vi "Memory Map to Messages.vi"(4 "Smallest Write Command Size":u32(ring)=4 items=["256-bytes"=256, "128-bytes"=128, "64-bytes"=64, "32-bytes"=32, "16-bytes"=16, "8-bytes"=8, "4-bytes"=4], 5 "Erase Block Size":u32(ring)=1024 items=["1024-bytes"=1024, "512-bytes"=512, "256-bytes"=256, "128-bytes"=128, "64-bytes"=64, "32-bytes"=32, "16-bytes"=16, "8-bytes"=8], 6 "Largest Write Command Size":u32(ring)=256 items=["256-bytes"=256, "128-bytes"=128, "64-bytes"=64, "32-bytes"=32, "16-bytes"=16, "8-bytes"=8], 7 "Empty Range Thld":i32=8, 8 "error in":errorcluster, 10 "Check Memory Block Size":u32(ring)=16 items=["1024-bytes"=1024, "512-bytes"=512, "256-bytes"=256, "128-bytes"=128, "64-bytes"=64, "32-bytes"=32, "16-bytes"=16, "8-bytes"=8], 11 "base path":path=path "C:/SCU Flash Application/ODX File/C70/FlashDrvRAM.s19") -> (0 "Error Out":errorcluster, 1 "read memory list":cluster{"Address":i32, "Data":u8[]}[](array[cluster]) {"Address" format="%x"}, 2 "erase addresses":u32[](array[numeric]) format="%x", 3 "Messages":cluster{"Address":i32, "Data":u8[]}[](array[cluster]) {"Address" format="%.0x"; "Data" format="%.0x"})   [LabVIEW 2018]
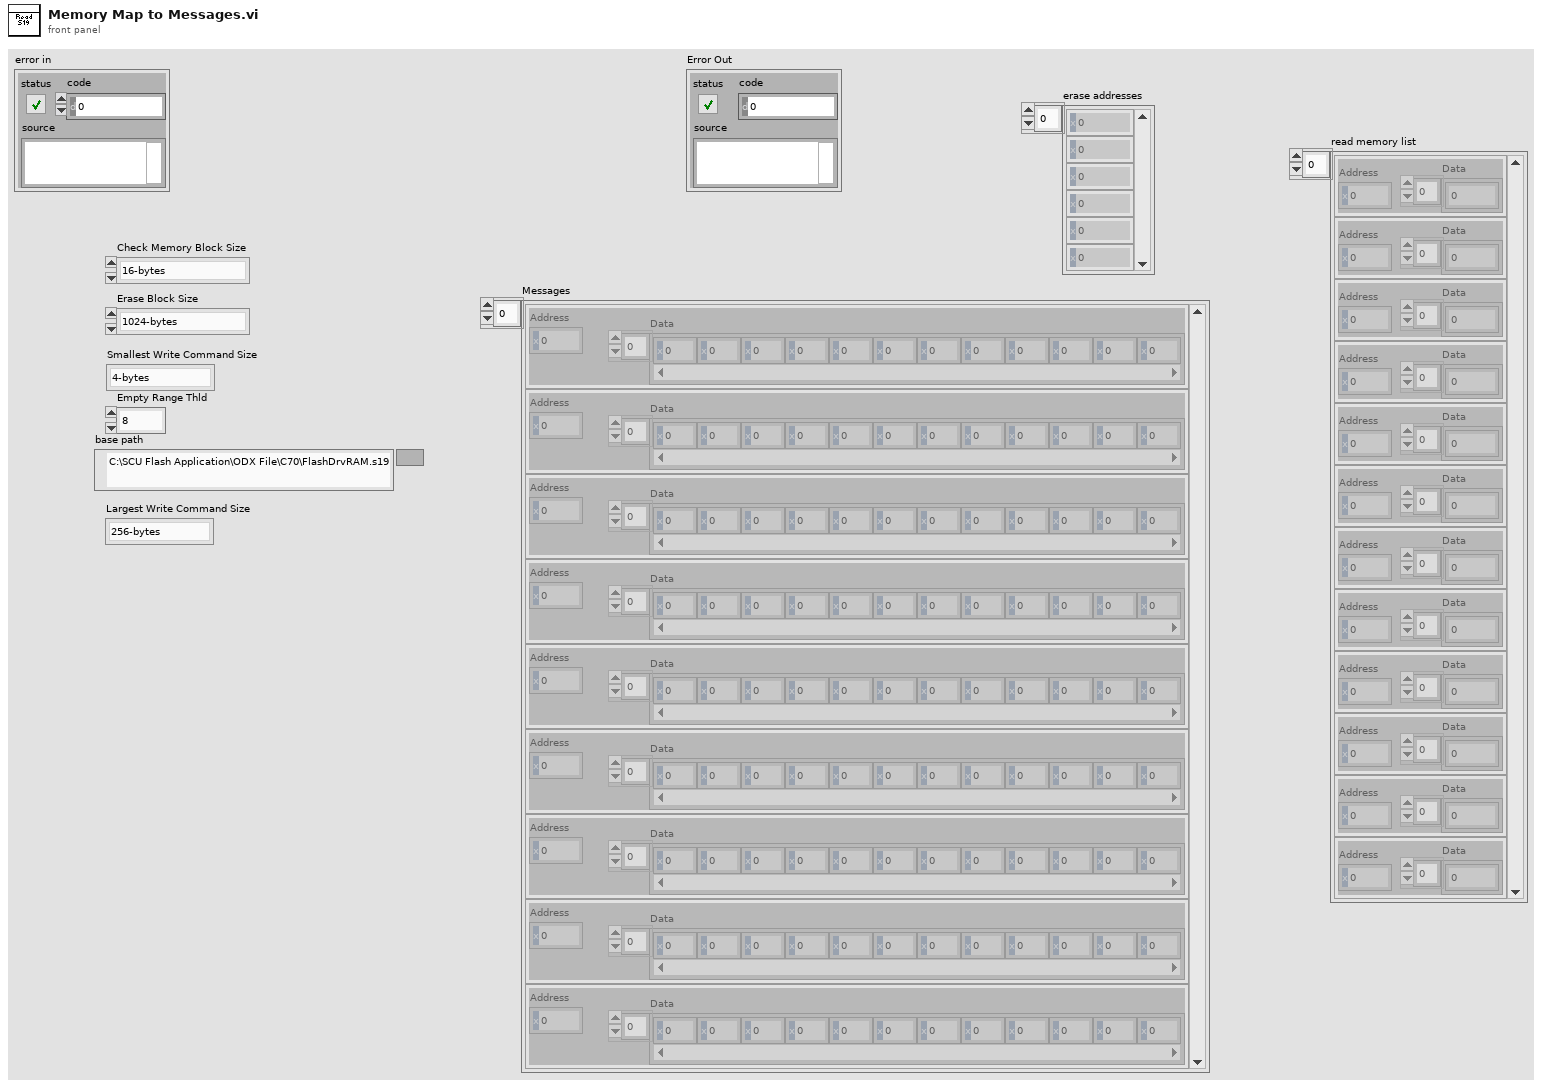
[diagram p1: front panel]
types:
  T1 = cluster{"Address":u32, "Data":u8[], "CheckSUM":u32}[]
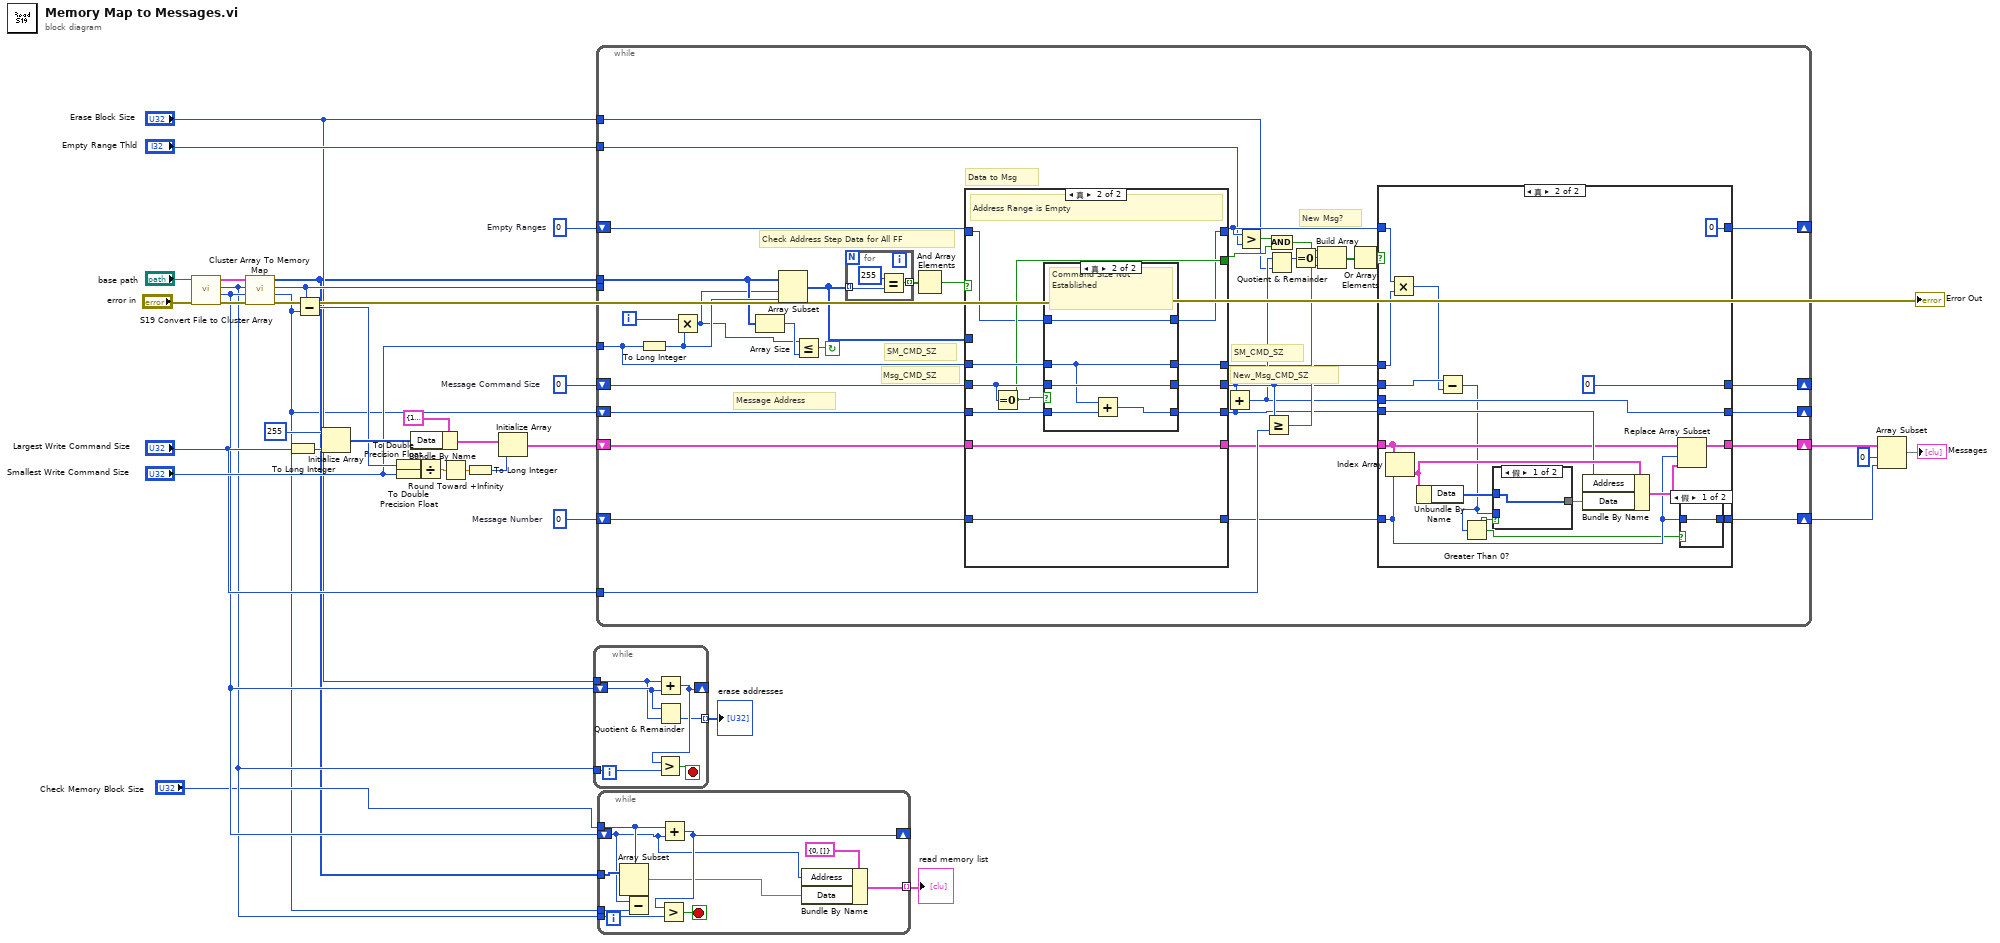
[diagram p0: block diagram]
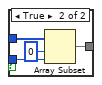
[diagram p3: hidden frame]
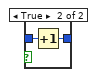
[diagram p4: hidden frame]
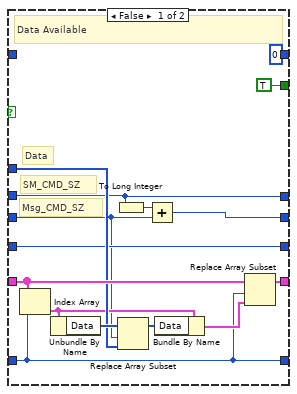
[diagram p5: hidden frame]
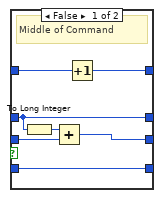
[diagram p6: hidden frame]
diagram:
  w19 = 0  # Empty Ranges
  w20 = 0  # Message Command Size
  w22 = 0  # Message Number
  n1 = call "S19 Convert File to Cluster Array.vi"("error in"="error in", "base path"="base path") -> ("Error Out"=→"Error Out":errorcluster, "Address Min"=w7:u32, "Address Max"=w6:u32, "数组"=w1:T1)  [unwired: 6 in]
  n2 = call "Cluster Array To Memory Map.vi"("Address Min in"=w7, "Address Max in"=w6, "Array in"=w1) -> ("Address Min out"=w3:u32, "Address Max out"=w10:u32, "Array out"=w4:u8[])  [unwired: 6 in]
  n3 = To Long Integer(number="Largest Write Command Size") -> (32bit integer=w34:i32)
  n4 = Subtract(x=w10, y=w3) -> (x-y=w29:u32)
  n5 = Initialize Array(u8 255 ("element"), w34) -> (w31:u8[])
  n6 = To Double Precision Float(number=w29) -> (double precision float=w25:dbl)
  n7 = To Double Precision Float(number="Smallest Write Command Size") -> (double precision float=w24:dbl)
  n8 = Bundle By Name(cluster=cluster{"Address":i32, "Data":u8[]} {"Address"=16777215, "Data"=[]} ("Line Data"), "Data"=w31) -> (w30:cluster{"Address":i32, "Data":u8[]})
  n9 = Divide(x=w25, y=w24) -> (x/y=w28:dbl)
  n10 = Round Toward +Infinity(x=w28) -> (ceil(x): smallest int >= x=w27:dbl)
  n11 = To Long Integer(number=w27) -> (32bit integer=w26:i32)
  n12 = Initialize Array(w30, w26) -> (w23:cluster{"Address":i32, "Data":u8[]}[])
  n13 = while {
    tunnel: [w38] -> w8 mode=indexing
    shift-right: [w39] -> _
    shift-left: w7 -> [w37]
    tunnel: w6 -> [w40]
    tunnel: "Erase Block Size" -> [w36]
    stop <- w41 stop-if-true
    n14 = Add(x=w36, y=w37) -> (x+y=w39:u32)
    n15 = Greater?(x=w39, y=w40) -> (0:w41:bool)
    n16 = Quotient & Remainder(x=w37, y=w36) -> (floor(x/y)=w38:u32)  [unwired: 1 out]
  }
  "erase addresses" <- w8
  n17 = while {
    tunnel: w4 -> [w51]
    shift-right: [w60] -> w15
    shift-left: w23 -> [w76]
    shift-right: [w59] -> w16
    shift-left: w22 -> [w77]
    tunnel: w10 -> [_]
    tunnel: "Smallest Write Command Size" -> [w74]
    shift-right: [w62] -> _
    shift-left: w3 -> [w49]
    shift-right: [w58] -> _
    shift-left: w20 -> [w75]
    shift-right: [w56] -> _
    shift-left: w19 -> [w72]
    tunnel: "Largest Write Command Size" -> [w70]
    tunnel: "Empty Range Thld" -> [w43]
    tunnel: "Erase Block Size" -> [w42]
    i -> [w47]
    stop <- w53 continue-if-true
    # "New Msg?"
    # "Data to Msg"
    # "SM_CMD_SZ"
    # "New_Msg_CMD_SZ"
    # "Msg_CMD_SZ"
    # "SM_CMD_SZ"
    # "Message Address"
    # "Check Address Step Data for All FF"
    n18 = To Long Integer(number=w74) -> (32bit integer=w52:i32)
    n19 = Multiply(x=w47, y=w52) -> (x*y=w48:i32)
    n20 = Array Size(array=w51) -> (size(s)=w50:i32)
    n21 = Array Subset(array=w51, index=w48, length=w52) -> (w73:u8[])
    n22 = Less Or Equal?(x=w48, y=w50) -> (x <= y?=w53:bool)
    n23 = for {
      tunnel: w73 -> [w111] mode=indexing
      tunnel: [w112] -> w79 mode=indexing
      n24 = Equal?(x=u8 255, y=w111) -> (x = y?=w112:bool)
    }
    n25 = And Array Elements(Boolean array=w79) -> (logical AND=w78:bool)
    n26 = case shown="真" w78 {
      tunnel: w77 -> [w116 w136]
      tunnel: w49 -> [w119 w139]
      tunnel: w76 -> [w128 w137]
      tunnel: w75 -> [w118 w134]
      tunnel: w74 -> [w115 w138]
      tunnel: [w121 w133] -> w64
      tunnel: [w122 w137] -> w66
      tunnel: w73 -> [w126 _]
      tunnel: w72 -> [_ w130]
      tunnel: [0 w129] -> w55
      tunnel: [w116 w136] -> w65
      tunnel: [w119 w135] -> w63
      tunnel: [w115 w132] -> w57
      tunnel: [TRUE w131] -> w44
      frame False {
        # "Data"
        # "Msg_CMD_SZ"
        # "SM_CMD_SZ"
        # "Data Available"
        n27 = Index Array(array=w128, index=w116) -> (element=w125:cluster{"Address":i32, "Data":u8[]})
        n28 = Unbundle By Name(w125) -> ("Data"=w127:u8[])
        n29 = To Long Integer(number=w115) -> (32bit integer=w117:i32)
        n30 = Replace Array Subset(array=w127, new element=w126, index=w118) -> (w124:u8[])
        n31 = Add(x=w117, y=w118) -> (x+y=w121:i32)
        n32 = Bundle By Name(cluster=w125, "Data"=w124) -> (w123:cluster{"Address":i32, "Data":u8[]})
        n33 = Replace Array Subset(array=w128, new element=w123, index=w116) -> (w122:cluster{"Address":i32, "Data":u8[]}[])
      }
      frame True {
        # "Address Range is Empty"
        n34 = Equal To 0?(x=w134) -> (x = 0?=w131:bool)
        n35 = case shown="真" w131 {
          tunnel: w139 -> [w146 w151]
          tunnel: w138 -> [w142 w148]
          tunnel: [w146 w150] -> w135
          tunnel: w134 -> [w145 w149]
          tunnel: [w143 w149] -> w133
          tunnel: [w142 w148] -> w132
          tunnel: w130 -> [w141 w147]
          tunnel: [w140 w147] -> w129
          frame False {
            # "Middle of Command"
            n36 = To Long Integer(number=w142) -> (32bit integer=w144:i32)
            n37 = Add(x=w144, y=w145) -> (x+y=w143:i32)
            n38 = Increment(x=w141) -> (x+1=w140:i32)
          }
          frame True {
            # "Command Size Not Established"
            n39 = Add(x=w148, y=w151) -> (x+y=w150:u32)
          }
        }
      }
    }
    n40 = Add(x=w64, y=w63) -> (x+y=w61:u32)
    n41 = Greater?(x=w55, y=w43) -> (0:w45:bool)
    n42 = Greater Or Equal?(x=w64, y=w70) -> (x >= y?=w67:bool)
    n43 = And(x=w45, y=w44) -> (x .and. y?=w46:bool)
    n44 = Quotient & Remainder(x=w61, y=w42) -> (x-y*floor(x/y)=w71:u32)  [unwired: 1 out]
    n45 = Equal To 0?(x=w71) -> (x = 0?=w69:bool)
    n46 = Build Array(w46, w69, w67) -> (w54:bool[])
    n47 = Or Array Elements(Boolean array=w54) -> (logical OR=w68:bool)
    n48 = case shown="真" w68 {
      tunnel: w66 -> [w81 w96]
      tunnel: w65 -> [w80 w94]
      tunnel: w64 -> [w83 w88]
      tunnel: w63 -> [w82 w99]
      tunnel: [w82 w98] -> w62
      tunnel: w61 -> [_ w98]
      tunnel: [w81 w95] -> w60
      tunnel: [w80 w93] -> w59
      tunnel: [w83 0 ("Message Command Size")] -> w58
      tunnel: w57 -> [_ w90]
      tunnel: [w84 0] -> w56
      tunnel: w55 -> [w84 w89]
      frame False {
      }
      frame True {
        n49 = Index Array(array=w96, index=w94) -> (element=w101:cluster{"Address":i32, "Data":u8[]})
        n50 = Multiply(x=w89, y=w90) -> (x*y=w87:u32)
        n51 = Unbundle By Name(w101) -> ("Data"=w102:u8[])
        n52 = Subtract(x=w88, y=w87) -> (x-y=w86:u32)
        n53 = Greater Than 0?(x=w86) -> (x > 0?=w85:bool)
        n54 = case shown="假" w85 {
          tunnel: w102 -> [w103 w107]
          tunnel: [w103 w105] -> w100
          tunnel: w86 -> [_ w104]
          frame False {
          }
          frame True {
            n55 = Array Subset(array=w107, index=0, length=w104) -> (w105:u8[])
          }
        }
        n56 = Bundle By Name(cluster=w101, "Address"=w99, "Data"=w100) -> (w97:cluster{"Address":i32, "Data":u8[]})
        n57 = Replace Array Subset(array=w96, new element=w97, index=w94) -> (w95:cluster{"Address":i32, "Data":u8[]}[])
        n58 = case shown="假" w85 {
          tunnel: w94 -> [w108 w110]
          tunnel: [w108 w109] -> w93
          frame False {
          }
          frame True {
            n59 = Increment(x=w110) -> (x+1=w109:i32)
          }
        }
      }
    }
  }
  n60 = while {
    shift-right: [w160] -> _
    shift-left: w7 -> [w152]
    tunnel: w6 -> [w161]
    tunnel: "Check Memory Block Size" -> [w154]
    tunnel: w4 -> [w159]
    tunnel: w3 -> [w155]
    tunnel: [w153] -> w2 mode=indexing
    stop <- w162 stop-if-true
    n61 = Subtract(x=w152, y=w155) -> (x-y=w156:u32)
    n62 = Array Subset(array=w159, index=w156, length=w154) -> (w157:u8[])
    n63 = Add(x=w154, y=w152) -> (x+y=w160:u32)
    n64 = Greater?(x=w160, y=w161) -> (0:w162:bool)
    n65 = Bundle By Name(cluster=cluster{"Address":i32, "Data":u8[]} {"Address"=0, "Data"=[]} ("Line Data"), "Address"=w152, "Data"=w157) -> (w153:cluster{"Address":i32, "Data":u8[]})
  }
  "read memory list" <- w2
  n66 = Array Subset(array=w15, index=0, length=w16) -> (→"Messages":cluster{"Address":i32, "Data":u8[]}[])
